vi "OC2 Send command.vi"(0 "VISA resource name":refnum<visa-resource-name>, 1 "Command data":string, 2 "Command":string, 3 "error in (no error)":errorcluster, 4 "coms":bool) -> (5 "dup VISA resource name":refnum<visa-resource-name>, 6 "error out":errorcluster)   [LabVIEW 2009]
doc: "TCM Send command.vi\n\nLow level VI that sends data commands to the TCM\n\nCOPYRIGHT ELECTRON DYNAMICS LTD"
panel:
  out "return count":u32
  out "checksum":u8 format="%.0x"
  out "unsigned byte array":u8[](array[numeric])
  out "Data sent":string
  out "length":i32
  # "Send command"
  # "V1.02"
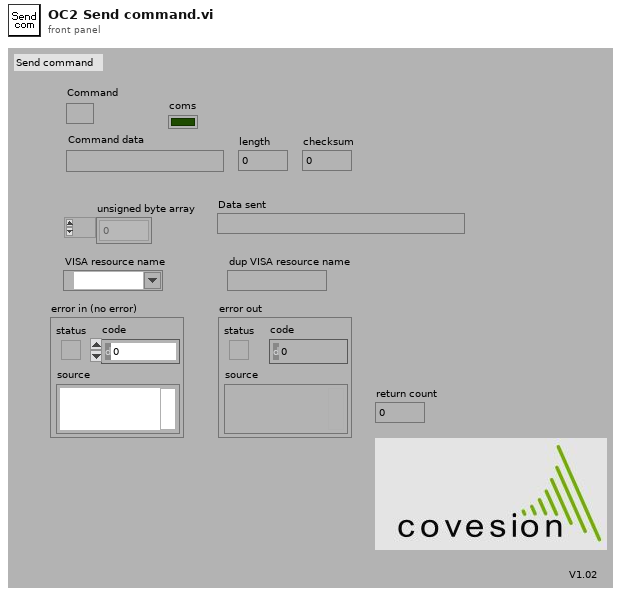
[diagram p1: front panel]
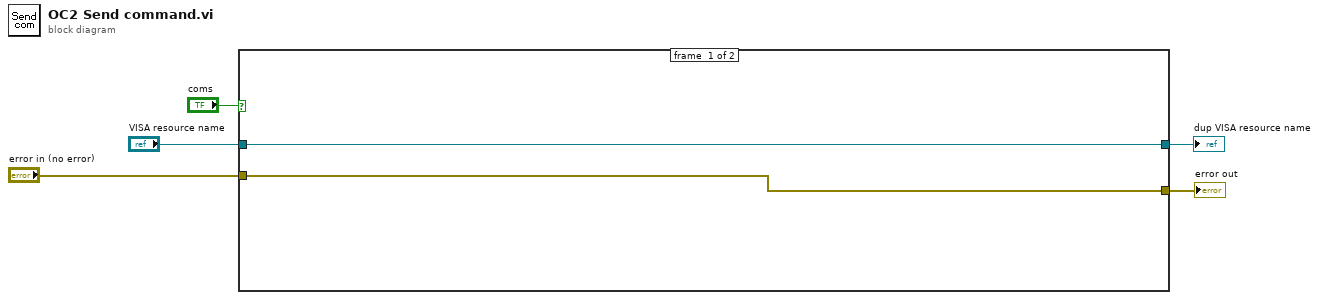
[diagram p0: block diagram]
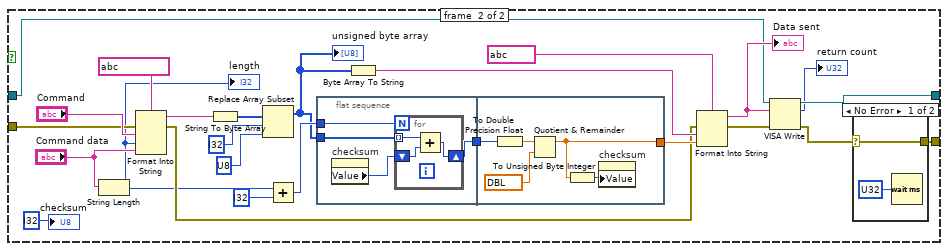
[diagram p2: hidden frame]
diagram:
  n1 = case shown="True" "coms" {
    tunnel: "VISA resource name" -> [w7 w17]
    tunnel: [w7 w16] -> w4
    tunnel: [w6 w8] -> w1
    tunnel: "error in (no error)" -> [w6 w15]
    frame #0 {
    }
    frame #1 {
      n2 = String Length(string="Command data") -> (length=w11:i32)
      "length" <- w11
      n3 = Format Into String(format string=string ?, error in=w15, "Command", w11, "Command data") -> (resulting string=w21:string, error out=w13:errorcluster)  [unwired: 1 in]
      n4 = String To Byte Array(string=w21) -> (unsigned byte array=w20:u8[])
      n5 = Replace Array Subset(array=w20, new element=u8 ?, index=i32 ?) -> (w19:u8[])
      "unsigned byte array" <- w19
      n6 = Add(x=w11, y=i32 ?) -> (x+y=w27:i32)
      n7 = flat-sequence {
        tunnel: w27 -> [w38]
        tunnel: w19 -> [w39]
        tunnel: [w37] -> w10
        tunnel: [w44] -> w22
        tunnel: w10 -> [w46]
        frame #0 {
          n8 = property on="checksum" class="DigNum (strict)"() -> ("Value"=w36:u8)  [unwired: 2 in, 2 out]
          n9 = for {
            N: w38 -> [_]
            tunnel: w39 -> [w42] mode=indexing
            shift-right: [w41] -> w37
            shift-left: w36 -> [w40]
            n10 = Add(x=w42, y=w40) -> (x+y=w41:u8)
          }
        }
        frame #1 {
          n11 = To Double Precision Float(number=w46) -> (double precision float=w45:dbl)
          n12 = Quotient & Remainder(x=w45, y=dbl ?) -> (x-y*floor(x/y)=w44:dbl)  [unwired: 1 out]
          n13 = To Unsigned Byte Integer(number=w44) -> (unsigned 8bit integer=w43:u8)
          n14 = property on="checksum" class="DigNum (strict)"("Value"=w43) -> ()  [unwired: 2 in, 2 out]
        }
      }
      n15 = Byte Array To String(unsigned byte array=w19) -> (string=w23:string)
      n16 = Format Into String(format string=string ?, error in=w13, w23, w22) -> (resulting string=w18:string, error out=w12:errorcluster)  [unwired: 1 in]
      "Data sent" <- w18
      n17 = VISA Write(VISA resource name=w17, write buffer=w18, error in (no error)=w12) -> (VISA resource name out=w16:refnum<visa-resource-name>, return count=→"return count":u32, error out=w9:errorcluster)
      n18 = case shown="No Error" w9 {
        selector: w9 -> [w34 w35]
        tunnel: [w34 w35] -> w8
        frame #0 {
          n19 = Wait (ms)(milliseconds to wait=u32 ?) -> ()  [unwired: 1 out]
        }
        frame #1 {
        }
      }
      "checksum" <- i32 ? ("checksum")
    }
  }
  "dup VISA resource name" <- w4
  "error out" <- w1
